vi "Validate Channels.vi"(7 "Channels Enum Variant":variant, 8 "error in (no error)":errorcluster, 11 "Channel Names":string[](array[string])) -> (0 "error out":errorcluster, 3 "Index Array":u16[](array[numeric]))   [LabVIEW 2021]
uses:
  <vilib>/Utility/VariantDataType/VariantType.lvlib
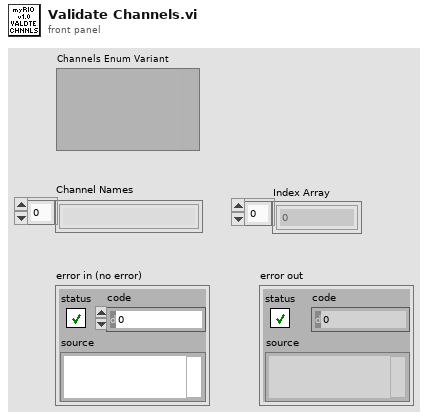
[diagram p1: front panel]
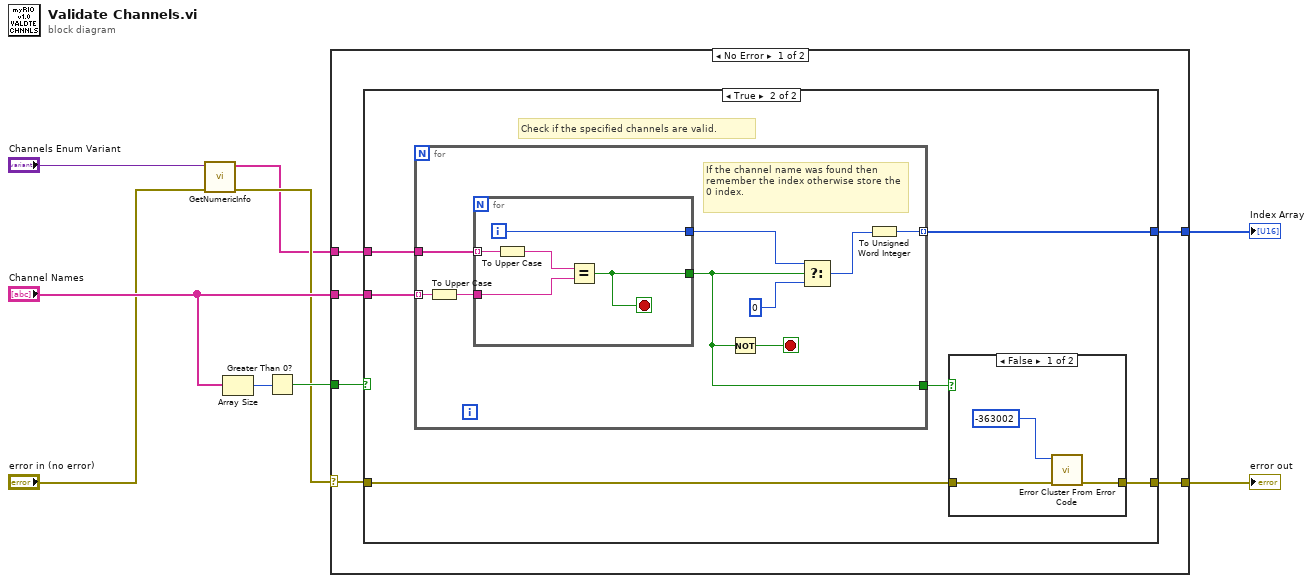
[diagram p0: block diagram]
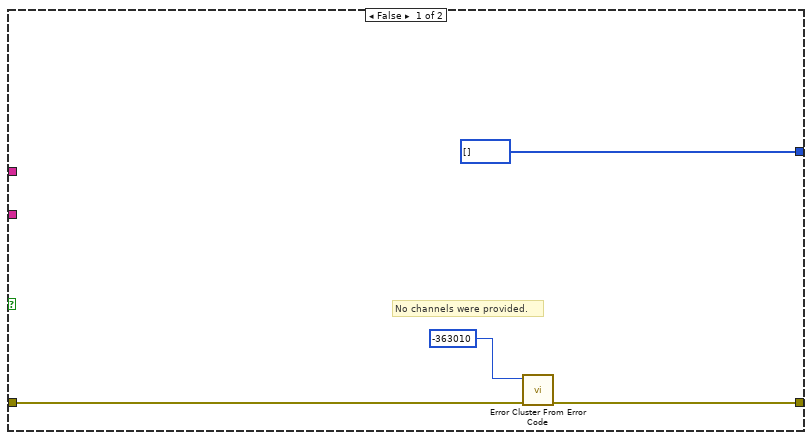
[diagram p2: hidden frame]
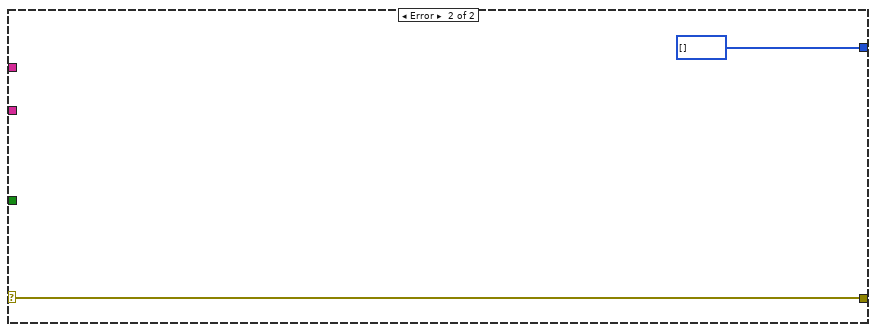
[diagram p4: hidden frame]
diagram:
  n1 = call <vilib>:"GetNumericInfo.vi"("error in (no error)"="error in (no error)", "Variant"="Channels Enum Variant") -> ("error out"=w2:errorcluster, "EnumNames"=w1:string[])  [unwired: 6 in, 2 out]
  n2 = Array Size(array="Channel Names") -> (size(s)=w6:i32)
  n3 = Greater Than 0?(x=w6) -> (x > 0?=w5:bool)
  n4 = case shown="No Error" w2 {
    selector: w2 -> [w10 w45]
    tunnel: [w15 w45] -> w9
    tunnel: w1 -> [w14 _]
    tunnel: [w13 u16[] []] -> w8
    tunnel: "Channel Names" -> [w12 _]
    tunnel: w5 -> [w11 _]
    frame No Error {
      n5 = case shown="True" w11 {
        tunnel: [w17 w25] -> w15
        tunnel: w10 -> [w18 w24]
        tunnel: w14 -> [_ w23]
        tunnel: [u16[] [] w22] -> w13
        tunnel: w12 -> [_ w21]
        frame False {
          # "No channels were provided."
          n6 = call <vilib>:"Error Cluster From Error Code.vi"("error in (no error)"=w18, "error code (0)"=-363010) -> ("error out"=w17:errorcluster)  [unwired: 7 in]
        }
        frame True {
          # "Check if the specified channels are valid."
          n7 = for {
            tunnel: w21 -> [w35] mode=indexing
            tunnel: w23 -> [w38]
            tunnel: [w36] -> w22 mode=indexing
            tunnel: [w33] -> w20
            stop <- w34 stop-if-true
            # "If the channel name was found then remember the index otherwise store the 0 index."
            n8 = To Upper Case(1:w35) -> (0:w37:string)
            n9 = for {
              tunnel: w38 -> [w43] mode=indexing
              tunnel: w37 -> [w41]
              tunnel: [w40] -> w33
              tunnel: [w39] -> w32
              i -> [w39]
              stop <- w40 stop-if-true
              n10 = To Upper Case(1:w43) -> (0:w42:string)
              n11 = Equal?(x=w42, y=w41) -> (x = y?=w40:bool)
            }
            n12 = Not(x=w33) -> (.not. x?=w34:bool)
            n13 = Select(t=w32, s=w33, f=0) -> (s? t:f=w30:i32)
            n14 = To Unsigned Word Integer(number=w30) -> (unsigned 16bit integer=w36:u16)
          }
          n15 = case shown="False" w20 {
            tunnel: w24 -> [w27 w29]
            tunnel: [w26 w29] -> w25
            frame False {
              n16 = call <vilib>:"Error Cluster From Error Code.vi"("error in (no error)"=w27, "error code (0)"=-363002) -> ("error out"=w26:errorcluster)  [unwired: 7 in]
            }
            frame True {
            }
          }
        }
      }
    }
    frame Error {
    }
  }
  "error out" <- w9
  "Index Array" <- w8
